vi "FPGA_target_reinitialise_memory_data.vi"(0 "number_cmds":u32) -> ()   [LabVIEW 2014]
doc: "this VI re-initializes the counter variables of the \"jump\" commands"
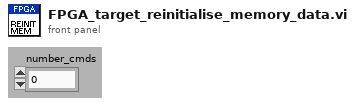
[diagram p1: front panel]
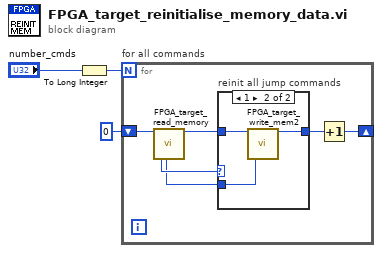
[diagram p0: block diagram]
diagram:
  n1 = To Long Integer(number="number_cmds") -> (32bit integer=w2:i32)
  n2 = for "for all commands" {
    N: w2 -> [_]
    shift-right: [w6] -> _
    shift-left: u32 0 -> [w9]
    n3 = call "FPGA_target_read_memory.vi"("addr_in"=w9) -> ("data_mem0"=w5:u8, "data_mem1"=w4:u32, "addr_dup"=w8:u32)  [unwired: 13 in, 3 out]
    n4 = case "reinit all jump commands" shown="1" w5 {
      tunnel: w8 -> [w10 w13]
      tunnel: [w10 w12] -> w7
      tunnel: w4 -> [_ w11]
      frame 0, Default {
      }
      frame 1 {
        n5 = call "FPGA_target_write_mem2.vi"("mem_addr_in"=w13, "mem_data"=w11) -> ("mem_addr_out"=w12:u32)  [unwired: 17 in]
      }
    }
    n6 = Increment(x=w7) -> (x+1=w6:u32)
  }
